vi "Write.vi"(8 "error in (no error)":errorcluster, 10 "Numeric":dbl, 11 "Numeric Array in":refnum<class "Double Float Array 1D.lvclass">) -> (0 "error out":errorcluster, 3 "Numeric Array out":refnum<class "Double Float Array 1D.lvclass">)   [LabVIEW 2021, in "Variable.lvlib" / "Double Float Array 1D.lvclass"]
uses:
  Double Float Array 1D.lvclass
  C:/Users/Tim/Documents/LabVIEW/2021/Data Classes/Source/Element/Vector Parent/Vector Parent.lvclass
  Element/Vector Parent/Vector Parent.lvclass/Vector Parent.ctl
  Double Float Array 1D.lvclass/Double Float Array 1D.ctl
  Element/Vector Parent/Properties/Read Index.vi
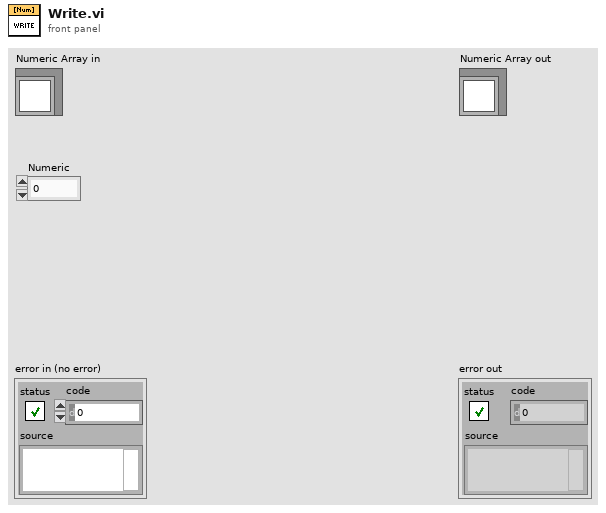
[diagram p1: front panel]
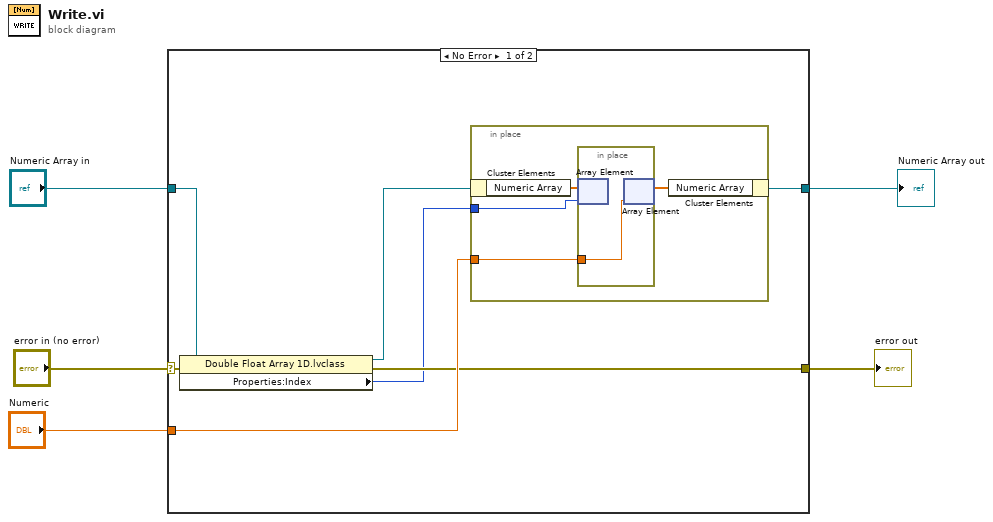
[diagram p0: block diagram]
diagram:
  n1 = case shown="No Error" "error in (no error)" {
    selector: "error in (no error)" -> [w10 w19]
    tunnel: [w8 w19] -> w4
    tunnel: "Numeric Array in" -> [w9 w18]
    tunnel: "Numeric" -> [w12 _]
    tunnel: [w11 w18] -> w1
    frame No Error {
      n2 = property class="Double Float Array 1D.lvclass"(reference=w9, error in=w10) -> (reference out=w7:refnum<class "Double Float Array 1D.lvclass">, error out=w8:errorcluster, "Properties:Index"=w6:i32)
      n3 = in-place {
        in-place-border: w6 -> [w15]
        in-place-border: w12 -> [w14]
        n4 = in-place-cluster #1(w7) -> ("Numeric Array"=w16:dbl[])
        n5 = in-place {
          in-place-border: w14 -> [w17]
          n6 = in-place-array #2(w16, w15) -> ()  [unwired: 1 out]
          n7 = in-place-array #2(w17) -> (w13:dbl[])  [unwired: 1 out]
        }
        n8 = in-place-cluster #1("Numeric Array"=w13) -> (w11:refnum<class "Double Float Array 1D.lvclass">)
      }
    }
    frame Error {
    }
  }
  "error out" <- w4
  "Numeric Array out" <- w1
